vi "XLP80_EIP_Init.vi"(8 "err in":errorcluster caption="error") -> (0 "err out":errorcluster caption="error")   [LabVIEW 2021]
uses:
  XLP80_Globals/Globals_Settings_XLP80.vi
  XLP80_General_Libs/Kirschenhofer_Libs/KH EthernetIP 17.19/KH_EthernetIP_Globals.vi
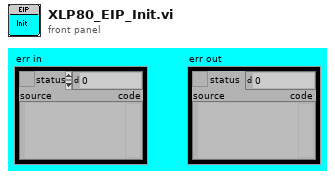
[diagram p1: front panel]
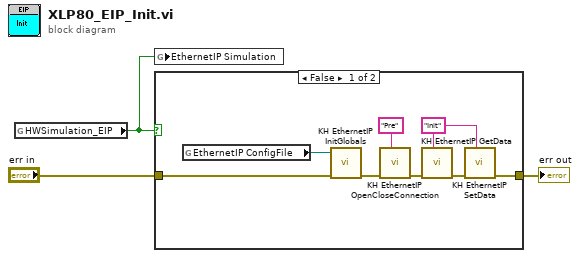
[diagram p0: block diagram]
diagram:
  n1 = global read "Globals_Settings_XLP80.vi" "HWSimulation_EIP"() -> (w1:bool)
  n2 = global write "KH_EthernetIP_Globals.vi" "EthernetIP Simulation"(w1) -> ()
  n3 = case shown="False" w1 {
    tunnel: [w11 w12] -> w3
    tunnel: "err in" -> [w10 w12]
    frame False {
      w5 = "Init" ("Function")
      n4 = global read "Globals_Settings_XLP80.vi" "EthernetIP ConfigFile"() -> (w4:path)
      n5 = call "KH EthernetIP InitGlobals.vi"("err in"=w10, "Config File"=w4) -> ("err out"=w8:errorcluster)  [unwired: 9 in]
      n6 = call "KH EthernetIP OpenCloseConnection.vi"("Function"="Pre", "error in"=w8) -> ("error out"=w7:errorcluster)  [unwired: 9 in]
      n7 = call "KH EthernetIP GetData.vi"("Function"=w5, "error in"=w7) -> ("error out"=w6:errorcluster)  [unwired: 8 in, 1 out]
      n8 = call "KH EthernetIP SetData.vi"("Function"=w5, "error in"=w6) -> ("error out"=w11:errorcluster)  [unwired: 7 in, 2 out]
    }
    frame True {
    }
  }
  "err out" <- w3
